vi "Launch Asynchronous Action.vi"(8 "error in (no error)":errorcluster, 9 "Message Data":variant, 10 "Message":string, 11 "Asynchronous Action In":refnum<class "Asynchronous Action.lvclass">) -> (0 "error out":errorcluster, 3 "Asynchronous Action Out":refnum<class "Asynchronous Action.lvclass">)   [LabVIEW 2020, in "Asynchronous Action.lvclass"]
doc: "Launches an asynchronous helper loop. Multiple helper loops may be launched using multiple calls to this VI. The Message and Message Data provided to this VI will be available in the Helper Action.vi once running."
uses:
  Asynchronous Action.lvclass
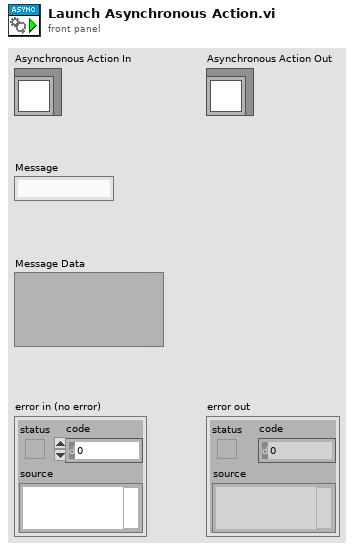
[diagram p1: front panel]
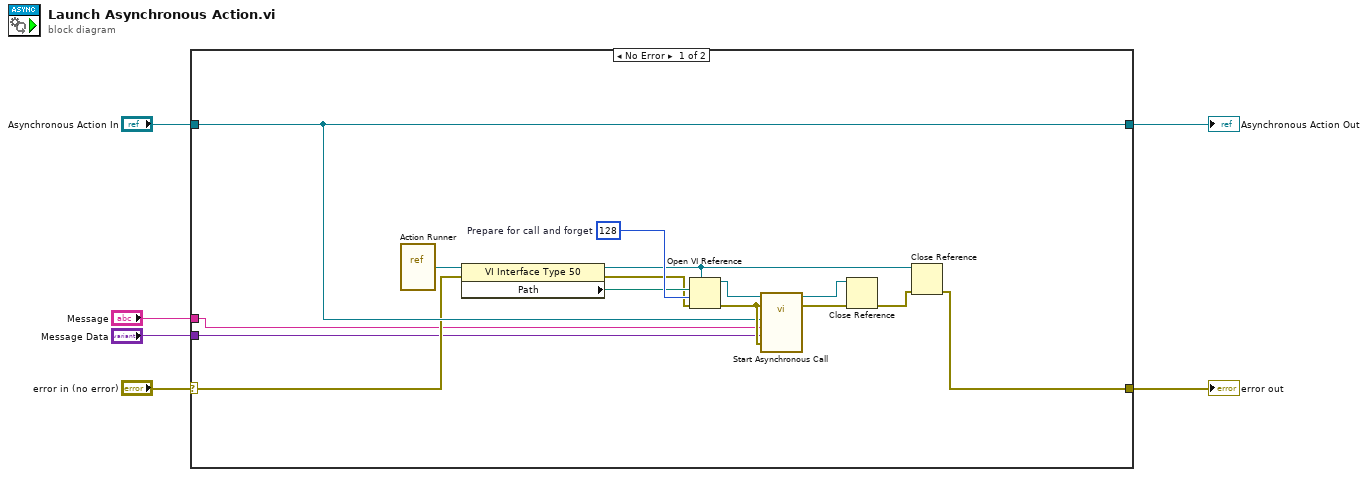
[diagram p0: block diagram]
diagram:
  n1 = case shown="No Error" "error in (no error)" {
    selector: "error in (no error)" -> [w10 w23]
    tunnel: [w12 w23] -> w5
    tunnel: [w11 w22] -> w4
    tunnel: "Asynchronous Action In" -> [w11 w22]
    tunnel: "Message" -> [w9 _]
    tunnel: "Message Data" -> [w8 _]
    frame No Error {
      w18 = 128  # Prepare for call and forget
      n2 = vi-ref "Action Runner.vi"() -> (w19:refnum<vi>)
      n3 = property class="VI Interface Type 50"(reference=w19, error in=w10) -> (reference out=w7:refnum<vi>, error out=w14:errorcluster, "Path"=w16:path)
      n4 = Open VI Reference(type specifier VI Refnum (for type only)=w7, vi path=w16, options=w18, error in (no error)=w14) -> (vi reference=w17:refnum<vi>, error out=w15:errorcluster)  [unwired: 2 in]
      n5 = call-by-ref "Start Asynchronous Call"(reference=w17, error in=w15, 8:"error in (no error)"=w15, "Message Data"=w8, "Message"=w9, "Asynchronous Action In"=w11) -> (reference out=w21:refnum<vi>, error out=w20:errorcluster)  [unwired: 6 in, 2 out]
      n6 = Close Reference(reference=w21, error in (no error)=w20) -> (error out=w13:errorcluster)
      n7 = Close Reference(reference=w7, error in (no error)=w13) -> (error out=w12:errorcluster)
    }
    frame Error {
    }
  }
  "error out" <- w5
  "Asynchronous Action Out" <- w4
